vi "LvHostsEdit4cRIO_SUB_HostInfo_Global.vi"() -> ()   [LabVIEW 2014]
uses:
  LvHostsEdit4cRIO_Rsc_HostInfo_Typedef.ctl
panel:
  in  "HostInfo[]":T1[](array[typedef])=[{"enable"=TRUE, "IP"="127.0.0.1", "Hostname"="localhost", "Alias"="", "Comment"=""}]
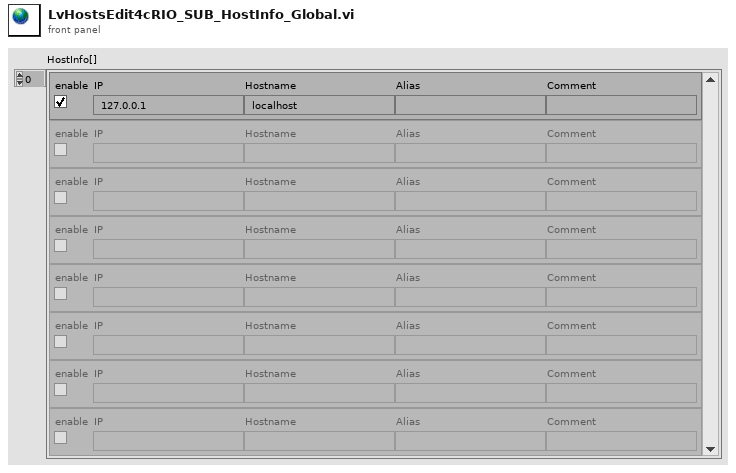
[diagram p1: front panel]
types:
  T1 = typedef "LvHostsEdit4cRIO_Rsc_HostInfo_Typedef.ctl" = cluster{"enable":bool, "IP":string, "Hostname":string, "Alias":string, "Comment":string}
diagram:
